vi "Create Log.vi"(11 "Model":string) -> (3 "refnum out":refnum<file>, 5 "path":path)   [LabVIEW 2021]
panel:
  out "error out":errorcluster
  in  "error in":errorcluster
  in  "DirectoryPath":string="c:\\Data\\"
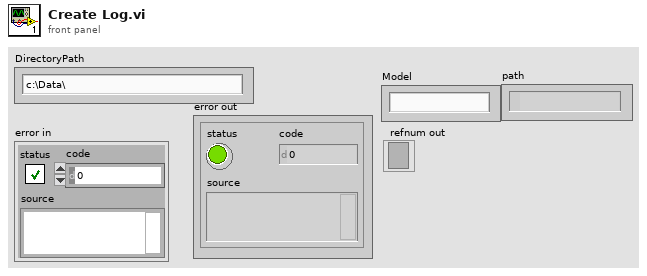
[diagram p1: front panel]
types:
  T1 = enum16{"open", "replace", "create", "open or create", "replace or create", "replace or create with confirmation"}
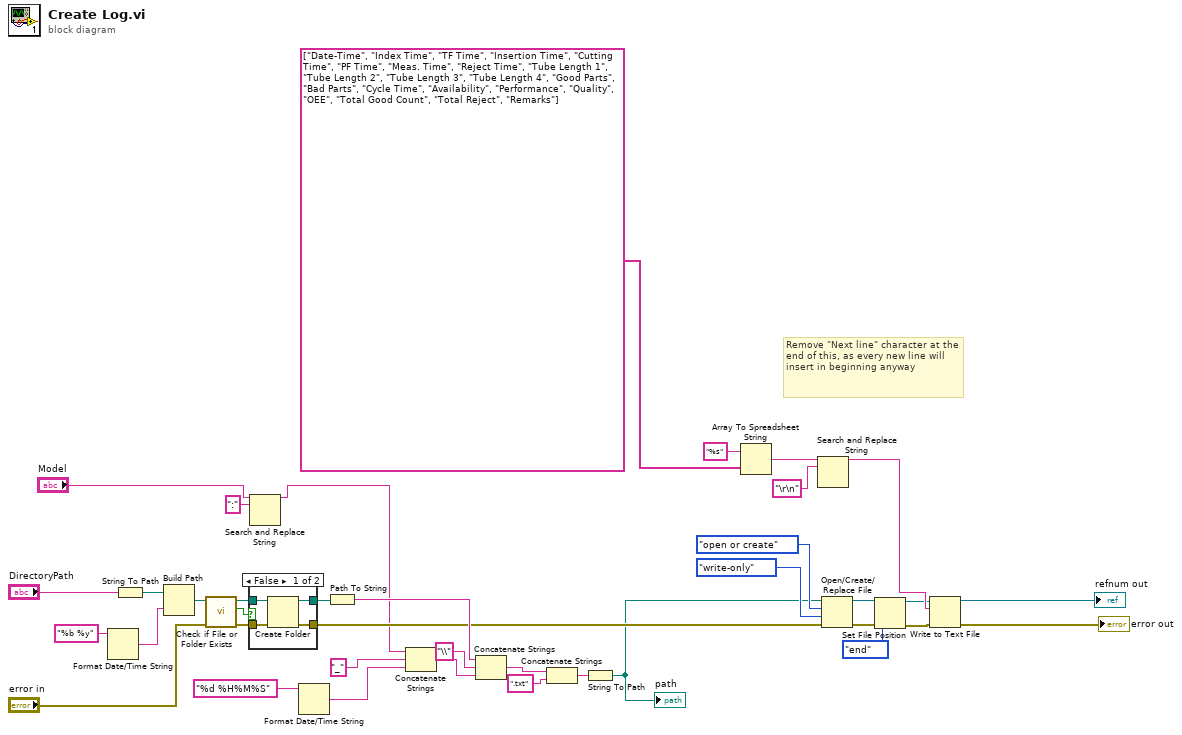
[diagram p0: block diagram]
diagram:
  # "Remove \"Next line\" character at the end of this, as every new line will insert in beginning anyway"
  n1 = Format Date/Time String(time format string (%c)="%b %y") -> (date/time string=w34:string)  [unwired: 2 in]
  n2 = String To Path(string="DirectoryPath") -> (path=w33:path)
  n3 = Build Path(base path=w33, name or relative path=w34) -> (appended path=w29:path)
  n4 = call <vilib>:"Check if File or Folder Exists.vi"("error in (no error)"="error in", "path"=w29) -> ("error out"=w25:errorcluster, "file or folder exists?"=w15:bool, "dup path"=w30:path)  [unwired: 7 in]
  n5 = case shown="False" w15 {
    tunnel: w30 -> [w42 w44]
    tunnel: [w41 w44] -> w32
    tunnel: w25 -> [w40 w43]
    tunnel: [w39 w43] -> w21
    frame False {
      n6 = Create Folder(path (use dialog)=w42, error in=w40) -> (created path=w41:path, error out=w39:errorcluster)  [unwired: 1 in, 1 out]
    }
    frame True {
    }
  }
  n7 = Search and Replace String(input string="Model", search string=":") -> (result string=w1:string)  [unwired: 6 in, 3 out]
  n8 = Format Date/Time String(time format string (%c)="%d %H%M%S") -> (date/time string=w23:string)  [unwired: 2 in]
  n9 = Path To String(path=w32) -> (string=w22:string)
  n10 = Concatenate Strings(w1, "_" ("string"), w23) -> (w27:string)
  n11 = Concatenate Strings(w22, "\\" ("string"), w27) -> (w28:string)
  n12 = Concatenate Strings(w28, ".txt" ("string")) -> (w5:string)
  n13 = String To Path(string=w5) -> (path=w6:path)
  "path" <- w6
  n14 = Array To Spreadsheet String(array=string[] ["Date-Time", "Index Time", "TF Time", "Insertion Time", "Cutting Time", "PF Time", "Meas. Time", "Reject Time", "Tube Length 1", "Tube Length 2", "Tube Length 3", "Tube Length 4", "Good Parts", "Bad Parts", "Cycle Time", "Availability", "Performance", "Quality", "OEE", "Total Good Count", "Total Reject", "Remarks"] ("Step Constants"), 3:"%s" ("format string")) -> (spreadsheet string=w18:string)  [unwired: 1 in]
  n15 = Search and Replace String(input string=w18, search string="\r\n" ("replace string (\"\")")) -> (result string=w17:string)  [unwired: 6 in, 3 out]
  n16 = Open/Create/Replace File(file path (use dialog)=w6, error in=w21, operation (0:open)=T1."open or create", access (0:read/write)=enum16{"read/write", "read-only", "write-only"}."write-only") -> (refnum out=w10:refnum<file>, error out=w11:errorcluster)  [unwired: 2 in, 1 out]
  n17 = Set File Position(refnum=w10, from (0:start)=enum16{"start", "end", "current"}."end", error in=w11) -> (refnum out=w9:refnum<file>, error out=w8:errorcluster)  [unwired: 1 in]
  n18 = Write to Text File(file (use dialog)=w9, text=w17, error in=w8) -> (refnum out=→"refnum out":refnum<file>, error out=→"error out":errorcluster)  [unwired: 1 in, 1 out]
